vi "euclidean_distance_single.vi"(8 "Point 2 Y":sgl, 9 "Point 2 X":sgl, 10 "Point 1 Y":sgl, 11 "Point 1 X":sgl) -> (3 "Distance":sgl)   [LabVIEW 2019]
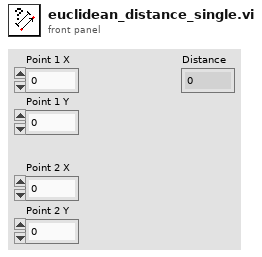
[diagram p1: front panel]
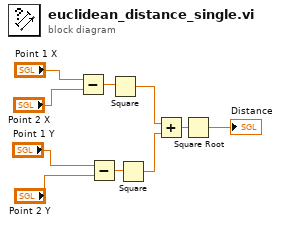
[diagram p0: block diagram]
diagram:
  n1 = Subtract(x="Point 1 X", y="Point 2 X") -> (x-y=w10:sgl)
  n2 = Subtract(x="Point 1 Y", y="Point 2 Y") -> (x-y=w9:sgl)
  n3 = Square(x=w10) -> (x^2=w8:sgl)
  n4 = Square(x=w9) -> (x^2=w7:sgl)
  n5 = Add(x=w8, y=w7) -> (x+y=w6:sgl)
  n6 = Square Root(x=w6) -> (sqrt(x)=→"Distance":sgl)
